vi "Get Positioner Error And Controller State Descriptions_libESP301.vi"(0 "Controller state":string, 4 "Positioner error":string) -> (1 "Color":u32(colorbox), 2 "Action name":string, 3 "Controller state description":string, 5 "IsReady?":bool, 6 "Positioner error boolean array":bool[][](array[boolean]), 7 "Positioner error description":string)   [LabVIEW 2019, in "Newport ESP301.lvlib"]
doc: "Decode the positioner error to an easier to use form."
uses:
  Newport ESP301.lvlib
panel:
  # "(ef)"
  # "(abcd)"
  # "a"
  # "D1: Char #"
  # "b"
  # "D2: Bit #"
  # "c"
  # "d"
  # "0    1    2    3"
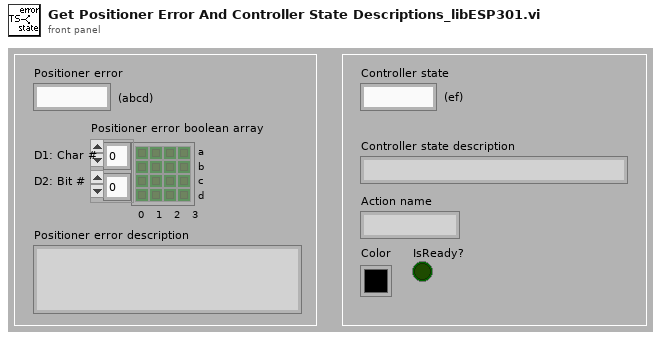
[diagram p1: front panel]
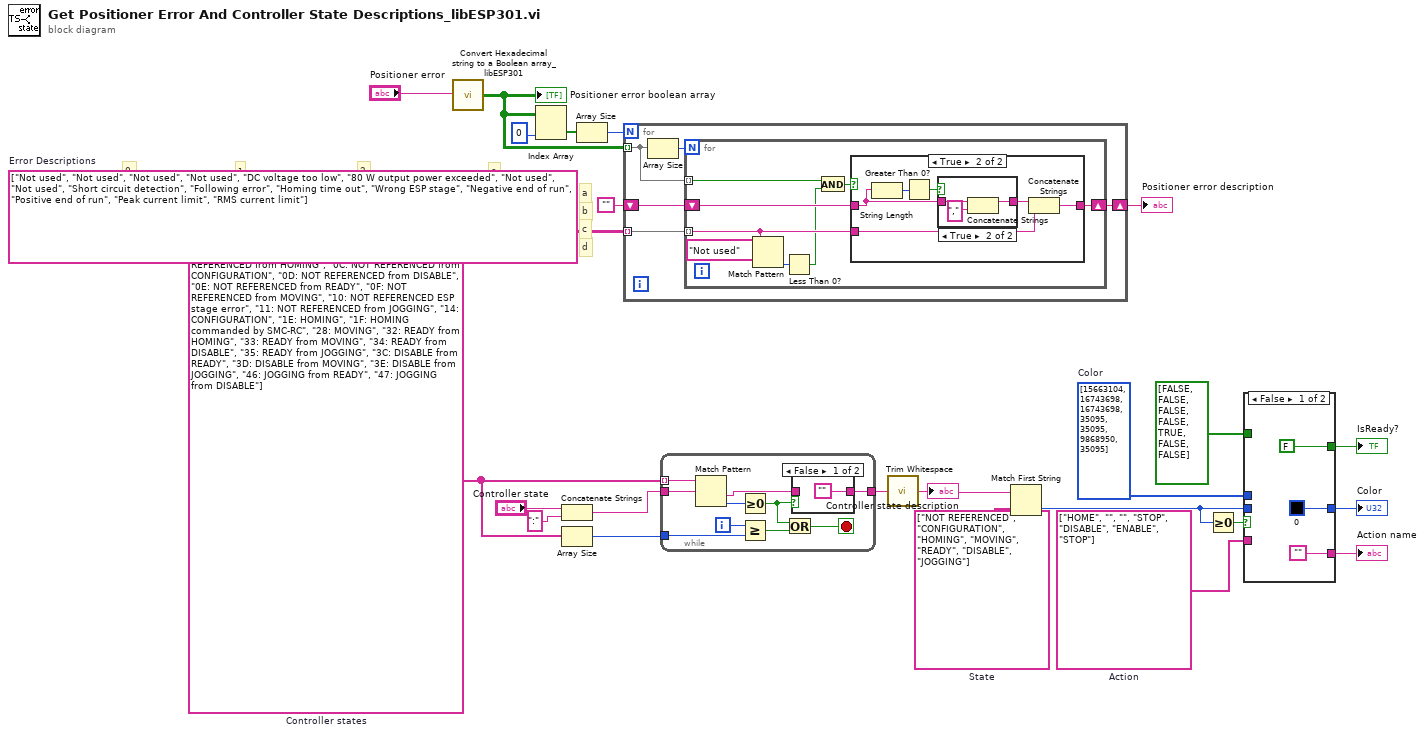
[diagram p0: block diagram]
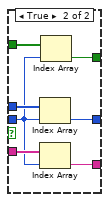
[diagram p2: hidden frame]
diagram:
  w4 = string[] ["HOME", "", "", "STOP", "DISABLE", "ENABLE", "STOP"]  # Action
  w8 = u32[] [15663104, 16743698, 16743698, 35095, 35095, 9868950, 35095]  # Color
  w9 = string[] ["NOT REFERENCED", "CONFIGURATION", "HOMING", "MOVING", "READY", "DISABLE", "JOGGING"]  # State
  w11 = string[][] [["Not used", "Not used", "Not used", "Not used"], ["DC voltage too low", "80 W output power exceeded", "Not used", "Not used"], ["Short circuit detection", "Following error", "Homing time out", "Wrong ESP stage"], ["Negative end of run", "Positive end of run", "Peak current limit", "RMS current limit"]]  # Error Descriptions
  w17 = string[] ["0A: NOT REFERENCED from reset", "0B: NOT REFERENCED from HOMING", "0C: NOT REFERENCED from CONFIGURATION", "0D: NOT REFERENCED from DISABLE", "0E: NOT REFERENCED from READY", "0F: NOT REFERENCED from MOVING", "10: NOT REFERENCED ESP stage error", "11: NOT REFERENCED from JOGGING", "14: CONFIGURATION", "1E: HOMING", "1F: HOMING commanded by SMC-RC", "28: MOVING", "32: READY from HOMING", "33: READY from MOVING", "34: READY from DISABLE", "35: READY from JOGGING", "3C: DISABLE from READY", "3D: DISABLE from MOVING", "3E: DISABLE from JOGGING", "46: JOGGING from READY", "47: JOGGING from DISABLE"]  # Controller states
  # "3"
  # "2"
  # "1"
  # "0"
  # "d"
  # "c"
  # "b"
  # "a"
  n1 = call "Convert Hexadecimal string to a Boolean array_libESP301.vi"("Hexadecimal String IN"="Positioner error") -> ("Boolean Array"=w12:bool[][])
  "Positioner error boolean array" <- w12
  n2 = Index Array(array=w12, index (col)=0 ("indice (ligne)")) -> (element=w21:bool[])  [unwired: 1 in]
  n3 = Concatenate Strings("Controller state", ":" ("chaîne")) -> (w14:string)
  n4 = Array Size(array=w17) -> (size(s)=w18:i32)
  n5 = Array Size(array=w21) -> (size(s)=w23:i32)
  n6 = for {
    N: w23 -> [_]
    tunnel: w11 -> [w27] mode=indexing
    tunnel: w12 -> [w28] mode=indexing
    shift-right: [w25] -> w19
    shift-left: "" -> [w26]
    n7 = Array Size(array=w28) -> (size(s)=w29:i32)
    n8 = for {
      N: w29 -> [_]
      tunnel: w28 -> [w31] mode=indexing
      tunnel: w27 -> [w35] mode=indexing
      shift-right: [w36] -> w25
      shift-left: w26 -> [w37]
      n9 = Match Pattern(string=w35, regular expression="Not used" ("chaîne faux")) -> (offset past match=w33:i32)  [unwired: 4 out]
      n10 = Less Than 0?(x=w33) -> (x < 0?=w30:bool)
      n11 = And(x=w31, y=w30) -> (x .and. y?=w32:bool)
      n12 = case shown="True" w32 {
        tunnel: w35 -> [_ w41]
        tunnel: w37 -> [w38 w42]
        tunnel: [w38 w39] -> w36
        frame False {
        }
        frame True {
          n13 = String Length(string=w42) -> (length=w44:i32)
          n14 = Greater Than 0?(x=w44) -> (x > 0?=w43:bool)
          n15 = case shown="True" w43 {
            tunnel: w42 -> [w45 w47]
            tunnel: [w45 w46] -> w40
            frame False {
            }
            frame True {
              n16 = Concatenate Strings(w47, ",") -> (w46:string)
            }
          }
          n17 = Concatenate Strings(w40, w41) -> (w39:string)
        }
      }
    }
  }
  "Positioner error description" <- w19
  n18 = while {
    tunnel: w18 -> [w57]
    tunnel: w17 -> [w56] mode=indexing
    tunnel: w14 -> [w51]
    tunnel: [w50] -> w13
    i -> [w58]
    stop <- w53 stop-if-true
    n19 = Match Pattern(string=w56, regular expression=w51) -> (after substring=w49:string, offset past match=w55:i32)  [unwired: 3 out]
    n20 = Greater Or Equal To 0?(x=w55) -> (x >= 0?=w52:bool)
    n21 = Greater Or Equal?(x=w58, y=w57) -> (x >= y?=w54:bool)
    n22 = Or(x=w52, y=w54) -> (x .or. y?=w53:bool)
    n23 = case shown="False" w52 {
      tunnel: ["" w60] -> w50
      tunnel: w49 -> [_ w60]
      frame False {
      }
      frame True {
      }
    }
  }
  n24 = call <vilib>:"Trim Whitespace.vi"("string"=w13) -> ("trimmed string"=w10:string)  [unwired: 1 in]
  "Controller state description" <- w10
  n25 = Match First String(2:w9, 3:w10) -> (0:w5:i32)  [unwired: 1 out]
  n26 = Greater Or Equal To 0?(x=w5) -> (x >= 0?=w6:bool)
  n27 = case shown="False" w6 {
    tunnel: w8 -> [_ w70]
    tunnel: [u32 0 ("Color") w69] -> w7
    tunnel: w5 -> [_ w66]
    tunnel: w4 -> [_ w68]
    tunnel: ["" w67] -> w3
    tunnel: bool[] [FALSE, FALSE, FALSE, FALSE, TRUE, FALSE, FALSE] -> [_ w65]
    tunnel: [FALSE w64] -> w1
    frame False {
    }
    frame True {
      n28 = Index Array(array=w70, index=w66) -> (element=w69:u32)
      n29 = Index Array(array=w68, index=w66) -> (element=w67:string)
      n30 = Index Array(array=w65, index=w66) -> (element=w64:bool)
    }
  }
  "Color" <- w7
  "Action name" <- w3
  "IsReady?" <- w1
